vi "rad_List Application Images.vi"(7 "App Image Temp Folder":path, 8 "error in (no error)":errorcluster, 11 "App Images Folder":path=path "C:/dev/Architectures/Reference Designs/Application Deployment and Replication/Application Deployment Utility/trunk/source/Application Images") -> (0 "error out":errorcluster, 2 "Application Images Infomration":T1[](array[typedef]))   [LabVIEW 2013]
doc: "This VI checks the specified folder for application images and returns a list of application images with information."
uses:
  TypeDefs/rad_AppImage Information.ctl
  TypeDefs/rad_Application Image Properties.ctl
  TypeDefs/rad_FPGA Properties.ctl
  TypeDefs/rad_FPGA Flash Properties.ctl
  rad_Globals.vi
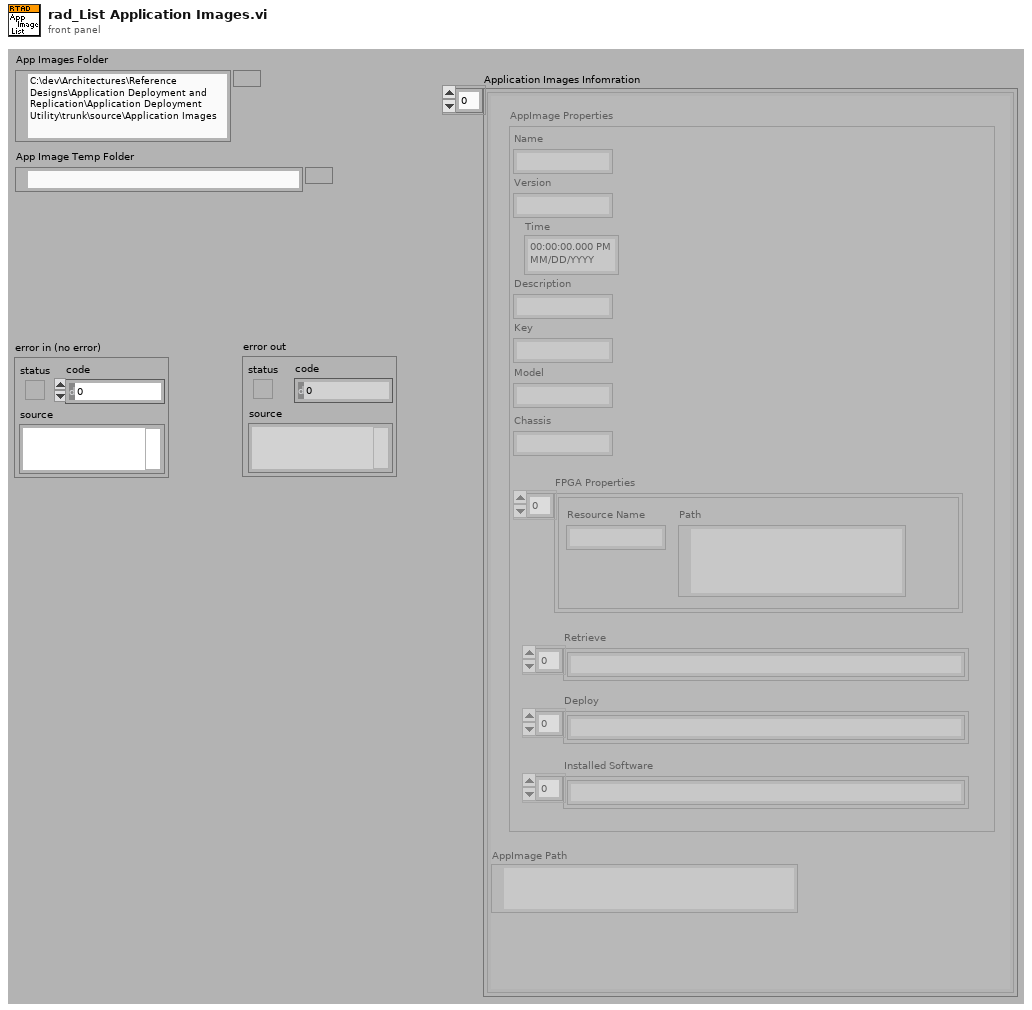
[diagram p1: front panel]
types:
  T1 = typedef "rad_AppImage Information.ctl" = cluster{"AppImage Properties":T2, "AppImage Path":path}
  T2 = typedef "rad_Application Image Properties.ctl" = cluster{"Name":string, "Version":string, "Time":timestamp, "Description":string, "Key":string, "Chassis":string, "FPGA Properties":T3, "Model":string, "Retrieve":string[], "Deploy":string[], "Installed Software":string[]}
  T3 = typedef "rad_FPGA Properties.ctl" = T4[]
  T4 = typedef "rad_FPGA Flash Properties.ctl" = cluster{"Resource Name":string, "Path":path}
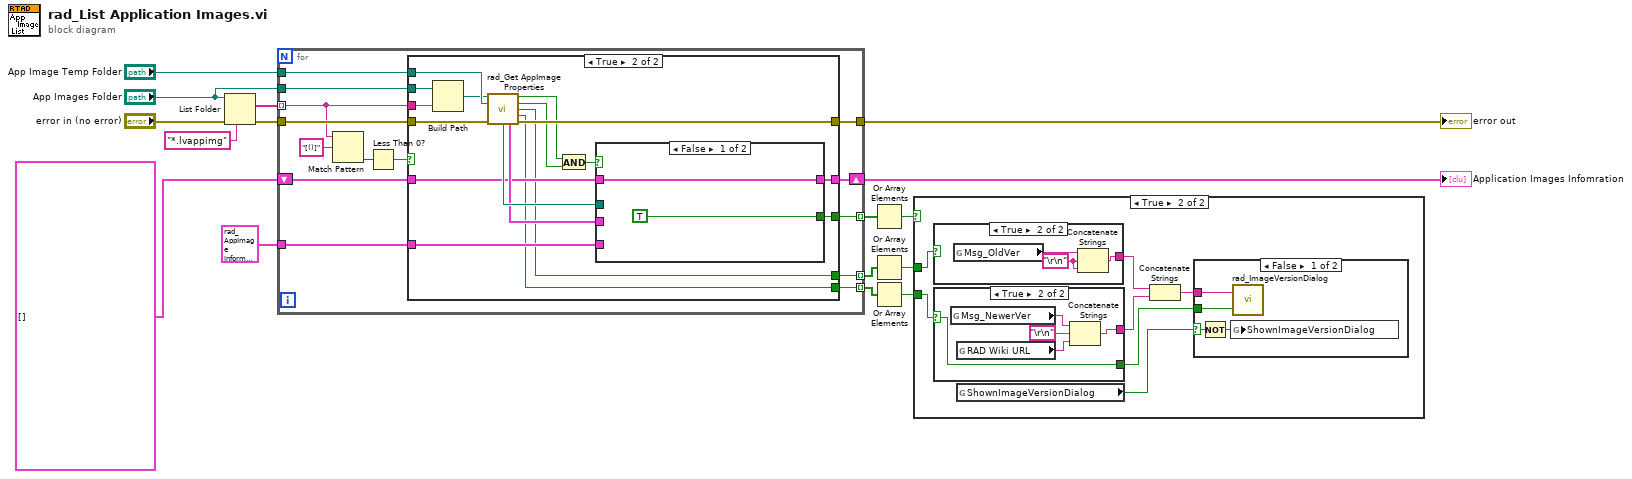
[diagram p0: block diagram]
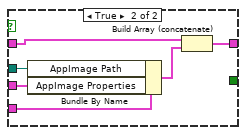
[diagram p7: hidden frame]
diagram:
  n1 = List Folder(path="App Images Folder", pattern="*.lvappimg", error in="error in (no error)") -> (filenames=w4:string[], error out=w6:errorcluster)  [unwired: 1 in, 2 out]
  n2 = for {
    tunnel: w4 -> [w20] mode=indexing
    tunnel: T1 {"AppImage Properties"={"Name"="", "Version"="", "Time"=timestamp(0 s since 1904-01-01), "Description"="", "Key"="", "Chassis"="", "FPGA Properties"=[], "Model"="", "Retrieve"=[], "Deploy"=[], "Installed Software"=[]}, "AppImage Path"=path ""} -> [w30]
    tunnel: w6 -> [w29]
    tunnel: [w28] -> w1
    tunnel: "App Image Temp Folder" -> [w22]
    shift-right: [w27] -> w2
    shift-left: T1[] [] -> [w26]
    tunnel: [w25] -> w11 mode=indexing
    tunnel: [w24] -> w10 mode=indexing
    tunnel: [w23] -> w13 mode=indexing
    tunnel: "App Images Folder" -> [w21]
    n3 = Match Pattern(string=w20, regular expression="[()]") -> (offset past match=w18:i32)  [unwired: 1 in, 3 out]
    n4 = Less Than 0?(x=w18) -> (x < 0?=w17:bool)
    n5 = case shown="True" w17 {
      tunnel: w30 -> [_ w49]
      tunnel: w29 -> [w32 w48]
      tunnel: [w32 w47] -> w28
      tunnel: [w31 w41] -> w27
      tunnel: w26 -> [w31 w40]
      tunnel: [_ w39] -> w25
      tunnel: [_ w38] -> w24
      tunnel: [_ w37] -> w23
      tunnel: w22 -> [_ w36]
      tunnel: w21 -> [_ w34]
      tunnel: w20 -> [_ w33]
      frame False {
      }
      frame True {
        n6 = Build Path(base path=w34, name or relative path=w33) -> (appended path=w35:path)
        n7 = call "rad_Get AppImage Properties.vi"("AppImage Path"=w35, "App Image Temp Folder"=w36, "error in (no error)"=w48) -> ("Supported"=w44:bool, "Current"=w43:bool, "Older"=w39:bool, "Newer"=w38:bool, "AppImage Path"=w46:path, "AppImage Properties"=w45:T2, "error out"=w47:errorcluster)  [unwired: 6 in]
        n8 = And(x=w44, y=w43) -> (x .and. y?=w42:bool)
        n9 = case shown="False" w42 {
          tunnel: w49 -> [_ w57]
          tunnel: w46 -> [_ w56]
          tunnel: w45 -> [_ w55]
          tunnel: [w51 w53] -> w41
          tunnel: w40 -> [w51 w52]
          tunnel: [TRUE _] -> w37
          frame False {
          }
          frame True {
            n10 = Bundle By Name(cluster=w57, "AppImage Path"=w56, "AppImage Properties"=w55) -> (w54:T1)
            n11 = Build Array (concatenate)(w52, w54) -> (w53:T1[])
          }
        }
      }
    }
  }
  "error out" <- w1
  "Application Images Infomration" <- w2
  n12 = Or Array Elements(Boolean array=w13) -> (logical OR=w12:bool)
  n13 = Or Array Elements(Boolean array=w11) -> (logical OR=w9:bool)
  n14 = Or Array Elements(Boolean array=w10) -> (logical OR=w8:bool)
  n15 = case shown="True" w12 {
    tunnel: w9 -> [_ w59]
    tunnel: w8 -> [_ w58]
    frame False {
    }
    frame True {
      n16 = case shown="True" w59 {
        tunnel: [_ w75] -> w62
        frame False {
        }
        frame True {
          w74 = "\r\n"
          n17 = global read "rad_Globals.vi" "Msg_OldVer"() -> (w76:string)
          n18 = Concatenate Strings(w76, w74, w74) -> (w75:string)
        }
      }
      n19 = case shown="True" w58 {
        selector: w58 -> [_ w71]
        tunnel: [_ w72] -> w63
        tunnel: [_ w71] -> w64
        frame False {
        }
        frame True {
          n20 = global read "rad_Globals.vi" "Msg_NewerVer"() -> (w73:string)
          n21 = global read "rad_Globals.vi" "RAD Wiki URL"() -> (w70:string)
          n22 = Concatenate Strings(w73, "\r\n", w70) -> (w72:string)
        }
      }
      n23 = global read "rad_Globals.vi" "ShownImageVersionDialog"() -> (w60:bool)
      n24 = Concatenate Strings(w62, w63) -> (w61:string)
      n25 = case shown="False" w60 {
        selector: w60 -> [w67 _]
        tunnel: w61 -> [w68 _]
        tunnel: w64 -> [w65 _]
        frame False {
          n26 = Not(x=w67) -> (.not. x?=w66:bool)
          n27 = global write "rad_Globals.vi" "ShownImageVersionDialog"(w66) -> ()
          n28 = call "rad_ImageVersionDialog.vi"("ShowUpgradeButton"=w65, "Message"=w68) -> ()  [unwired: 1 in]
        }
        frame True {
        }
      }
    }
  }
